vi "AMZ_S3_Create CommonHeaders String.vi"(11 "HTTP Headers in":T1[](array[typedef])) -> (2 "CommonHeaderValues":string, 3 "HTTP Headers":T1[](array[typedef]))   [LabVIEW 2015, in "LV Interface for Amazon S3.lvlib"]
doc: "Create the Common headers part of the String to Sign."
uses:
  LV Interface for Amazon S3.lvlib
  Typedefs/AMZ_S3_HTTP Header-Value pair.ctl
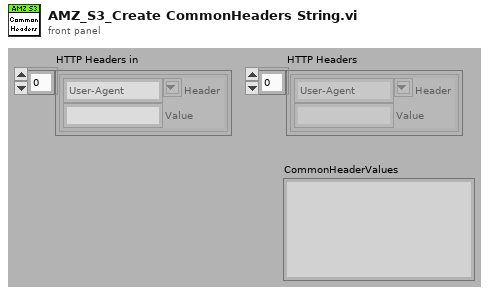
[diagram p1: front panel]
types:
  T1 = typedef "LV Interface for Amazon S3.lvlib/AMZ_S3_HTTP Header-Value pair.ctl" = cluster{"Header":string, "Value":string}
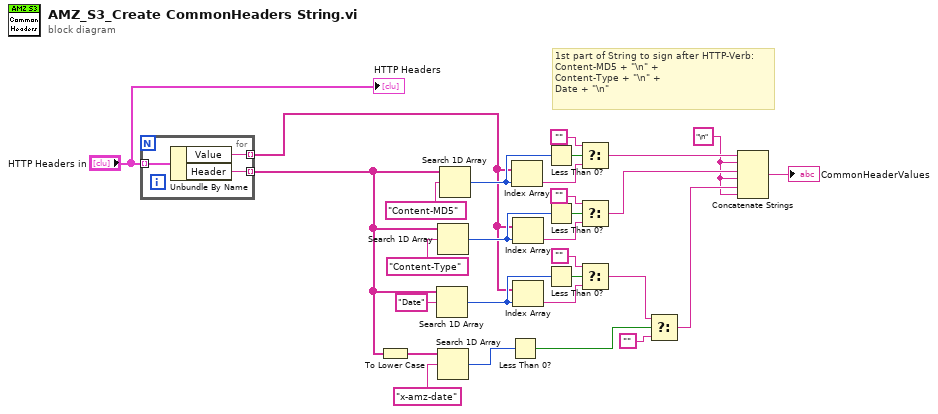
[diagram p0: block diagram]
diagram:
  w5 = "\n"
  # "1st part of String to sign after HTTP-Verb:\nContent-MD5 + \"\\n\" +\nContent-Type + \"\\n\" +\nDate + \"\\n\""
  n1 = for {
    tunnel: "HTTP Headers in" -> [w32] mode=indexing
    tunnel: [w31] -> w3 mode=indexing
    tunnel: [w30] -> w2 mode=indexing
    n2 = Unbundle By Name(w32) -> ("Value"=w30:string, "Header"=w31:string)
  }
  n3 = To Lower Case(string=w3) -> (all lower case string=w26:string[])
  n4 = Search 1D Array(1D array=w3, element="Date") -> (index of element=w21:i32)  [unwired: 1 in]
  n5 = Search 1D Array(1D array=w3, element="Content-Type") -> (index of element=w20:i32)  [unwired: 1 in]
  n6 = Search 1D Array(1D array=w26, element="x-amz-date") -> (index of element=w24:i32)  [unwired: 1 in]
  n7 = Search 1D Array(1D array=w3, element="Content-MD5") -> (index of element=w19:i32)  [unwired: 1 in]
  n8 = Less Than 0?(x=w24) -> (x < 0?=w23:bool)
  n9 = Index Array(array=w2, index=w19) -> (element=w12:string)
  n10 = Index Array(array=w2, index=w20) -> (element=w11:string)
  n11 = Index Array(array=w2, index=w21) -> (element=w10:string)
  n12 = Less Than 0?(x=w19) -> (x < 0?=w16:bool)
  n13 = Less Than 0?(x=w20) -> (x < 0?=w17:bool)
  n14 = Less Than 0?(x=w21) -> (x < 0?=w18:bool)
  n15 = Select(t="", s=w16, f=w12) -> (s? t:f=w8:string)
  n16 = Select(t="", s=w17, f=w11) -> (s? t:f=w7:string)
  n17 = Select(t="", s=w18, f=w10) -> (s? t:f=w9:string)
  n18 = Select(t=w9, s=w23, f="") -> (s? t:f=w6:string)
  n19 = Concatenate Strings(w8, w5, w7, w5, w6, w5) -> (→"CommonHeaderValues":string)
  "HTTP Headers" <- "HTTP Headers in"
